vi "Autonomous Independent.vi"   [LabVIEW 2013]
doc: "This VI is called when autonomous begins, and will automatically be terminated when autonomous ends. You can carry out timed or sensor driven robot movement independently without needing to return to the caller."
uses:
  <vilib>/Rock Robotics/WPI/SafetyOutput/WPI_SafetyOutputConfigMenu.ctl
  <vilib>/Rock Robotics/WPI/Solenoid/WPI_SolenoidValue.ctl
  Robot Global Data.vi
  <vilib>/Rock Robotics/WPI/RobotDrive/WPI_RobotDriveGetSetRefNum.vi
  <vilib>/Rock Robotics/WPI/Solenoid/WPI_SolenoidSetEnum.vi
  <vilib>/Rock Robotics/WPI/RobotDrive/WPI_RobotDriveArcadeDrive_Standard(NoSaturation).vi
panel:
  # "Be sure to right-click and choose Data Operations>>Make Current Value default if you want to save the array values with the VI"
types:
  T1 = typedef "WPI_SafetyOutputConfigMenu.ctl" = enum16{"Enable", "Disable"}
  T2 = typedef "WPI_RobotDriveDevRef.ctl" = cluster{"DevStatus":errorcluster, "Motors[]":T3[], "Square Inputs":bool, "Max Output":dbl, "Isochronous":bool}
  T3 = typedef "WPI_MotorControlDeviceRef.ctl" = cluster{"DeviceStatus":errorcluster, "Type":enum16{"PWM", "CAN"}, "PWM":cluster{"Digital Module":T4, "PWM Channel":T5, "DeadBand":T6}, "CAN":cluster{"Device Number":u8, "Control Mode":T7, "Semaphore":T8, "Max Vout":dbl}, "Invert":bool, "TransformRef":T9, "InvTransformRef":T9}
  T4 = typedef "FPGA_TypedefDigitalModule.ctl" = enum16{"Digital Module 1", "Digital Module 2"}
  T5 = typedef "FPGA_DIOPWMChannel.ctl" = enum8{"PWM 1", "PWM 2", "PWM 3", "PWM 4", "PWM 5", "PWM 6", "PWM 7", "PWM 8", "PWM 9", "PWM 10", "Invalid"}
  T6 = typedef "WPI_PWMDeadband.ctl" = cluster{"Name":string, "maxPositivePwm":i32, "minPositivePwm":i32, "centerPwm":i32, "maxNegativePwm":i32, "minNegativePwm":i32, "angularRange":u16}
  T7 = typedef "WPI_CANJaguar_ControlMode.ctl" = enum8{"Percent VBus", "Current", "Speed", "Position", "Voltage"}
  T8 = typedef "Semaphore RefNum" = refnum<k1>
  T9 = typedef "WPI_PWMTransform_ConPane.ctl" = refnum<vi>
  T10 = typedef "WPI_EncoderDevRef.ctl" = cluster{"DevStatus":errorcluster, "EncoderIndex":T11, "CounterIndex":T12, "DistancePerCount":dbl, "Decoding Type":T13}
  T11 = typedef "FPGA_EncoderIdx.ctl" = enum8{"Enc 0", "Enc 1", "Enc 2", "Enc 3", "Invalid"}
  T12 = typedef "FPGA_CounterCtrSystemIndex.ctl" = enum8{"Ctr 0", "Ctr 1", "Ctr 2", "Ctr 3", "Ctr 4", "Ctr 5", "Ctr 6", "Ctr 7", "Invalid"}
  T13 = typedef "WPI_EncoderType.ctl" = enum16{"1x", "2x", "4x"}
  T14 = typedef "WPI_SolenoidDevRef.ctl" = cluster{"DevStatus":errorcluster, "Solenoid Module":T15, "Forward Solenoid Channel":T16, "Reverse Solenoid Channel":T16}
  T15 = typedef "FPGA_TypedefSolenoidModule.ctl" = enum16{"Solenoid Module 1", "Solenoid Module 2"}
  T16 = typedef "WPI_SolenoidChannel.ctl" = enum8{"Solenoid 1", "Solenoid 2", "Solenoid 3", "Solenoid 4", "Solenoid 5", "Solenoid 6", "Solenoid 7", "Solenoid 8", "Invalid"}
  T17 = typedef "WPI_DigitalInputDevRef.ctl" = cluster{"DevStatus":errorcluster, "DIO Channel":T18, "Digital Module":T4}
  T18 = typedef "FPGA_DIOChannel.ctl" = enum8{"DIO 1", "DIO 2", "DIO 3", "DIO 4", "DIO 5", "DIO 6", "DIO 7", "DIO 8", "DIO 9", "DIO 10", "DIO 11", "DIO 12", "DIO 13", "DIO 14", "Invalid"}
  T19 = typedef "WPI_SolenoidValue.ctl" = enum16{"Off", "On", "Forward", "Reverse"}
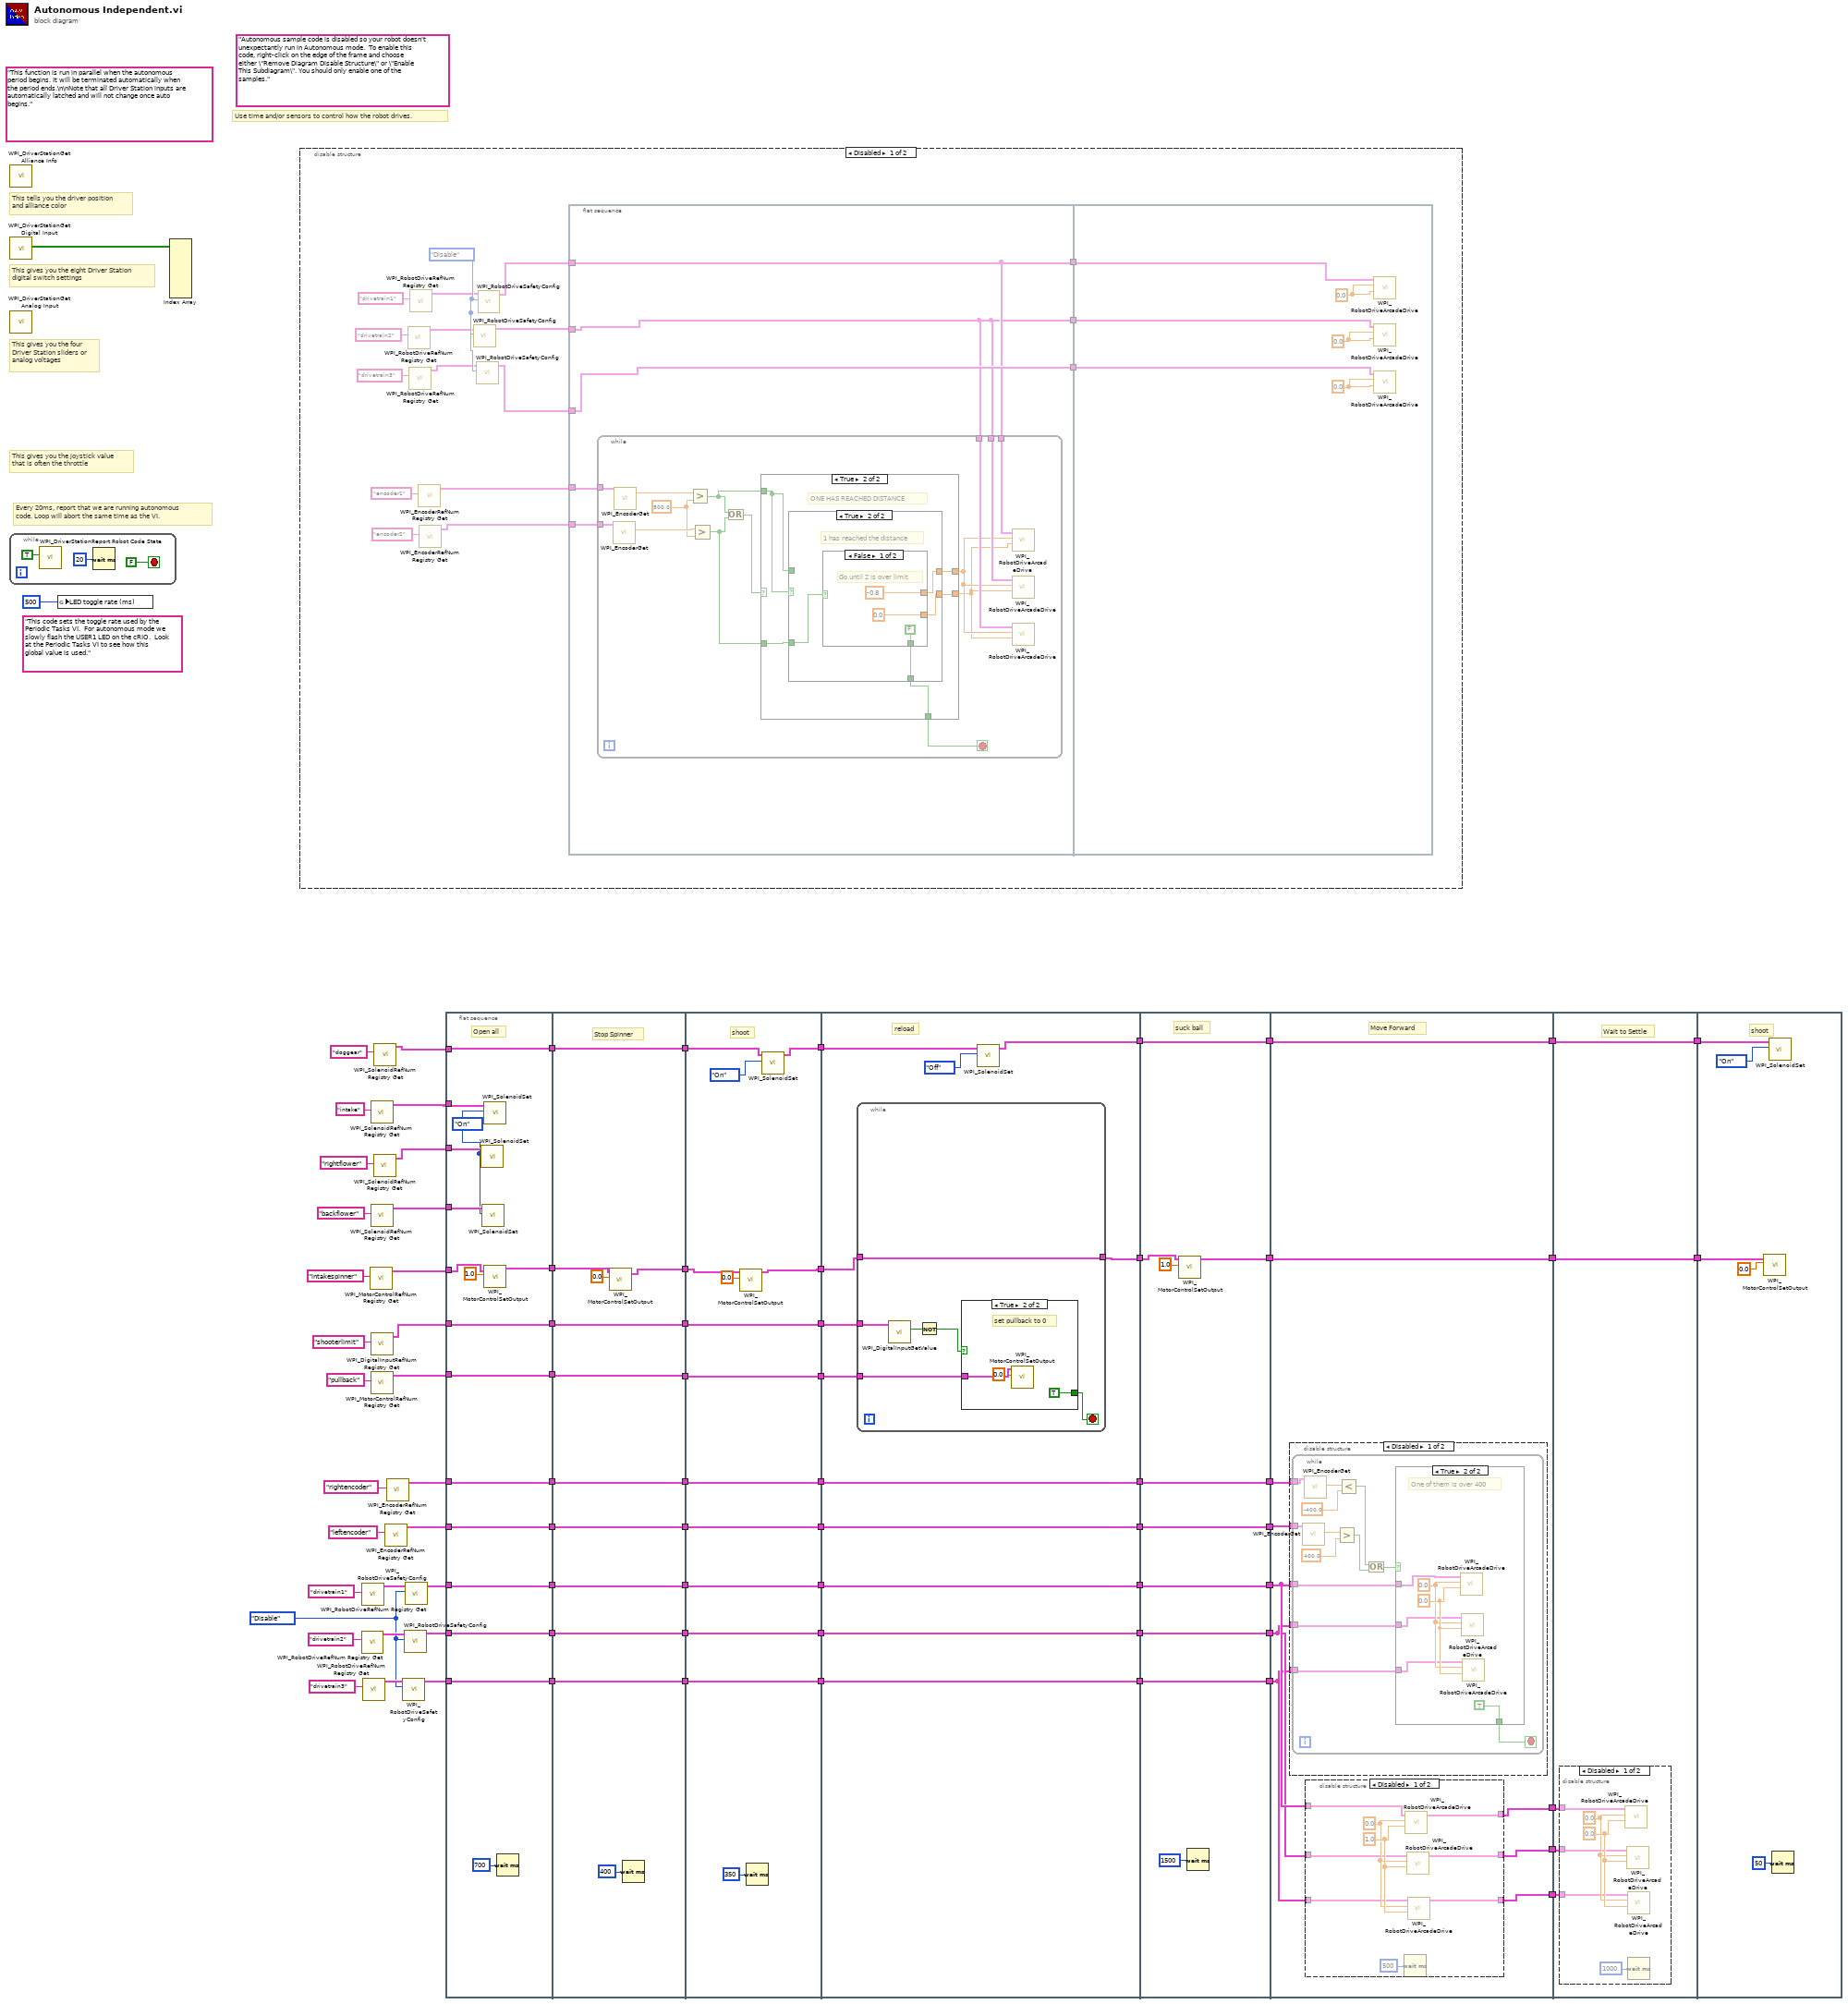
[diagram p0: block diagram]
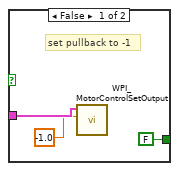
[diagram p2: hidden frame]
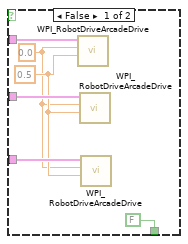
[diagram p4: hidden frame]
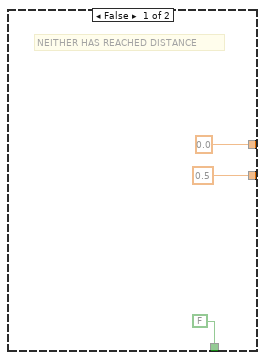
[diagram p7: hidden frame]
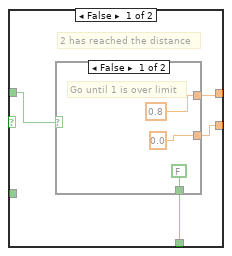
[diagram p8: hidden frame]
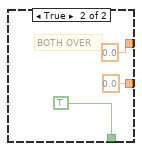
[diagram p9: hidden frame]
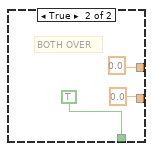
[diagram p10: hidden frame]
diagram:
  w38 = WPI_SafetyOutputConfigMenu."Disable" ("mode")
  (unwired) "This code sets the toggle rate used by the Periodic Tasks VI.  For autonomous mode we slowly flash the USER1 LED on the cRIO.  Look at the Periodic Tasks VI to see how this global value is used."
  (unwired) "Autonomous sample code is disabled so your robot doesn't unexpectantly run in Autonomous mode.  To enable this code, right-click on the edge of the frame and choose either \"Remove Diagram Disable Structure\" or \"Enable This Subdiagram\". You should only enable one of the samples."
  (unwired) "This function is run in parallel when the autonomous period begins. It will be terminated automatically when the period ends.\n\nNote that all Driver Station inputs are automatically latched and will not change once auto begins."
  # "Every 20ms, report that we are running autonomous\ncode. Loop will abort the same time as the VI."
  # "This gives you the joystick value\nthat is often the throttle"
  # "Use time and/or sensors to control how the robot drives."
  # "This tells you the driver position\nand alliance color"
  # "This gives you the eight Driver Station\ndigital switch settings"
  # "This gives you the four\nDriver Station sliders or\nanalog voltages"
  n1 = while {
    stop <- FALSE stop-if-true
    n2 = call <vilib>:"WPI_DriverStationReport Robot Code State.vi"("Autonomous"=TRUE) -> ()  [unwired: 10 in, 1 out]
    n3 = Wait (ms)(milliseconds to wait=u32 20) -> ()  [unwired: 1 out]
  }
  n4 = call <vilib>:"WPI_DriverStationGet Alliance Info.vi"() -> ()  [unwired: 12 out]
  n5 = call <vilib>:"WPI_DriverStationGet Digital Input.vi"() -> ("Driver Station Digital Input (1-8)"=w78:bool[])  [unwired: 11 out]
  n6 = call <vilib>:"WPI_DriverStationGet Analog Input.vi"() -> ()  [unwired: 12 out]
  n7 = global write "Robot Global Data.vi" "LED toggle rate (ms)"(u32 500 ("LED ms toggle rate")) -> ()
  n8 = Index Array(array=w78) -> ()  [unwired: 8 in, 8 out]
  n9 = disable-structure shown="Disabled" {
    frame Disabled {
      w92 = WPI_SafetyOutputConfigMenu."Disable" ("mode")
      n10 = call <vilib>:"WPI_RobotDriveRefNum Registry Get.vi"("refnum name"="drivetrain2") -> ("RobotDriveDevRef"=w90:T2)  [unwired: 9 in, 1 out]
      n11 = call <vilib>:"WPI_RobotDriveRefNum Registry Get.vi"("refnum name"="drivetrain3") -> ("RobotDriveDevRef"=w89:T2)  [unwired: 9 in, 1 out]
      n12 = call <vilib>:"WPI_RobotDriveRefNum Registry Get.vi"("refnum name"="drivetrain1") -> ("RobotDriveDevRef"=w91:T2)  [unwired: 9 in, 1 out]
      n13 = call <vilib>:"WPI_EncoderRefNum Registry Get.vi"("refnum name"="encoder1") -> ("EncoderDevRef"=w85:T10)  [unwired: 9 in, 1 out]
      n14 = call <vilib>:"WPI_EncoderRefNum Registry Get.vi"("refnum name"="encoder2") -> ("EncoderDevRef"=w84:T10)  [unwired: 9 in, 1 out]
      n15 = call <vilib>:"WPI_RobotDriveSafetyConfig.vi"("mode"=w92, "RobotDriveDevRef"=w90) -> ("RobotDriveDevRef"=w87:T2)  [unwired: 8 in, 1 out]
      n16 = call <vilib>:"WPI_RobotDriveSafetyConfig.vi"("mode"=w92, "RobotDriveDevRef"=w89) -> ("RobotDriveDevRef"=w86:T2)  [unwired: 8 in, 1 out]
      n17 = call <vilib>:"WPI_RobotDriveSafetyConfig.vi"("mode"=w92, "RobotDriveDevRef"=w91) -> ("RobotDriveDevRef"=w88:T2)  [unwired: 8 in, 1 out]
      n18 = flat-sequence {
        tunnel: w88 -> [w100]
        tunnel: w87 -> [w99]
        tunnel: w86 -> [w103]
        tunnel: [w100] -> w98
        tunnel: [w99] -> w97
        tunnel: [w103] -> w96
        tunnel: w85 -> [w102]
        tunnel: w84 -> [w101]
        tunnel: w98 -> [w151]
        tunnel: w97 -> [w150]
        tunnel: w96 -> [w149]
        frame #0 {
          n19 = while {
            tunnel: w102 -> [w117]
            tunnel: w101 -> [w116]
            tunnel: w100 -> [w109]
            tunnel: w99 -> [w108]
            tunnel: w99 -> [w107]
            stop <- w111 stop-if-true
            w113 = 500.0 ("y")
            n20 = call <vilib>:"WPI_EncoderGet.vi"("EncoderDevRef"=w116) -> ("Distance"=w114:dbl)  [unwired: 5 in, 5 out]
            n21 = call <vilib>:"WPI_EncoderGet.vi"("EncoderDevRef"=w117) -> ("Distance"=w115:dbl)  [unwired: 5 in, 5 out]
            n22 = Greater?(x=w115, y=w113) -> (0:w110:bool)
            n23 = Greater?(x=w114, y=w113) -> (0:w106:bool)
            n24 = Or(x=w110, y=w106) -> (x .or. y?=w112:bool)
            n25 = case shown="True" w112 {
              tunnel: [FALSE w123] -> w111
              tunnel: w110 -> [_ w124]
              tunnel: w106 -> [_ w125]
              tunnel: [0.0 ("y") w122] -> w105
              tunnel: [0.5 ("y") w121] -> w104
              frame False {
                # "NEITHER HAS REACHED DISTANCE"
              }
              frame True {
                # "ONE HAS REACHED DISTANCE"
                n26 = case shown="True" w124 {
                  tunnel: w125 -> [_ w139]
                  tunnel: w124 -> [w129 _]
                  tunnel: [w128 w138] -> w123
                  tunnel: [w127 w137] -> w122
                  tunnel: [w126 w136] -> w121
                  frame False {
                    # "2 has reached the distance"
                    n27 = case shown="False" w129 {
                      tunnel: [FALSE TRUE] -> w128
                      tunnel: [0.8 ("y") 0.0 ("y")] -> w127
                      tunnel: [0.0 ("y") 0.0 ("y")] -> w126
                      frame False {
                        # "Go until 1 is over limit"
                      }
                      frame True {
                        # "BOTH OVER"
                      }
                    }
                  }
                  frame True {
                    # "1 has reached the distance"
                    n28 = case shown="False" w139 {
                      tunnel: [FALSE TRUE] -> w138
                      tunnel: [-0.8 ("y") 0.0 ("y")] -> w137
                      tunnel: [0.0 ("y") 0.0 ("y")] -> w136
                      frame False {
                        # "Go until 2 is over limit"
                      }
                      frame True {
                        # "BOTH OVER"
                      }
                    }
                  }
                }
              }
            }
            n29 = call-poly <vilib>:"WPI_RobotDriveArcadeDrive.vi"("Y axis value"=w104, "X axis value"=w105, "RobotDriveDevRef"=w109) -> ()  [unwired: 6 in, 3 out]
            n30 = call-poly <vilib>:"WPI_RobotDriveArcadeDrive.vi"("Y axis value"=w104, "X axis value"=w105, "RobotDriveDevRef"=w108) -> ()  [unwired: 6 in, 3 out]
            n31 = call-poly <vilib>:"WPI_RobotDriveArcadeDrive.vi"("Y axis value"=w104, "X axis value"=w105, "RobotDriveDevRef"=w107) -> ()  [unwired: 6 in, 3 out]
          }
        }
        frame #1 {
          w146 = 0.0 ("Y axis value")
          w147 = 0.0 ("Y axis value")
          w148 = 0.0 ("Y axis value")
          n32 = call-poly <vilib>:"WPI_RobotDriveArcadeDrive.vi"("Y axis value"=w148, "X axis value"=w148, "RobotDriveDevRef"=w151) -> ()  [unwired: 6 in, 3 out]
          n33 = call-poly <vilib>:"WPI_RobotDriveArcadeDrive.vi"("Y axis value"=w147, "X axis value"=w147, "RobotDriveDevRef"=w150) -> ()  [unwired: 6 in, 3 out]
          n34 = call-poly <vilib>:"WPI_RobotDriveArcadeDrive.vi"("Y axis value"=w146, "X axis value"=w146, "RobotDriveDevRef"=w149) -> ()  [unwired: 6 in, 3 out]
        }
      }
    }
    frame Enabled {
    }
  }
  n35 = call <vilib>:"WPI_RobotDriveRefNum Registry Get.vi"("refnum name"="drivetrain2") -> ("RobotDriveDevRef"=w40:T2)  [unwired: 9 in, 1 out]
  n36 = call <vilib>:"WPI_RobotDriveRefNum Registry Get.vi"("refnum name"="drivetrain1") -> ("RobotDriveDevRef"=w41:T2)  [unwired: 9 in, 1 out]
  n37 = call <vilib>:"WPI_RobotDriveRefNum Registry Get.vi"("refnum name"="drivetrain3") -> ("RobotDriveDevRef"=w39:T2)  [unwired: 9 in, 1 out]
  n38 = call <vilib>:"WPI_MotorControlRefNum Registry Get.vi"("refnum name"="intakespinner") -> ("MotorControlDevRef"=w66:T3)  [unwired: 9 in, 1 out]
  n39 = call <vilib>:"WPI_SolenoidRefNum Registry Get.vi"("refnum name"="intake") -> ("SolenoidDevRef"=w70:T14)  [unwired: 9 in, 1 out]
  n40 = call <vilib>:"WPI_SolenoidRefNum Registry Get.vi"("refnum name"="backflower") -> ("SolenoidDevRef"=w68:T14)  [unwired: 9 in, 1 out]
  n41 = call <vilib>:"WPI_DigitalInputRefNum Registry Get.vi"("refnum name"="shooterlimit") -> ("DigitalInputDevRef"=w63:T17)  [unwired: 9 in, 1 out]
  n42 = call <vilib>:"WPI_MotorControlRefNum Registry Get.vi"("refnum name"="pullback") -> ("MotorControlDevRef"=w60:T3)  [unwired: 9 in, 1 out]
  n43 = call <vilib>:"WPI_SolenoidRefNum Registry Get.vi"("refnum name"="rightflower") -> ("SolenoidDevRef"=w69:T14)  [unwired: 9 in, 1 out]
  n44 = call <vilib>:"WPI_SolenoidRefNum Registry Get.vi"("refnum name"="doggear") -> ("SolenoidDevRef"=w75:T14)  [unwired: 9 in, 1 out]
  n45 = call <vilib>:"WPI_EncoderRefNum Registry Get.vi"("refnum name"="leftencoder") -> ("EncoderDevRef"=w34:T10)  [unwired: 9 in, 1 out]
  n46 = call <vilib>:"WPI_EncoderRefNum Registry Get.vi"("refnum name"="rightencoder") -> ("EncoderDevRef"=w36:T10)  [unwired: 9 in, 1 out]
  n47 = call <vilib>:"WPI_RobotDriveSafetyConfig.vi"("mode"=w38, "RobotDriveDevRef"=w39) -> ("RobotDriveDevRef"=w12:T2)  [unwired: 8 in, 1 out]
  n48 = call <vilib>:"WPI_RobotDriveSafetyConfig.vi"("mode"=w38, "RobotDriveDevRef"=w40) -> ("RobotDriveDevRef"=w22:T2)  [unwired: 8 in, 1 out]
  n49 = call <vilib>:"WPI_RobotDriveSafetyConfig.vi"("mode"=w38, "RobotDriveDevRef"=w41) -> ("RobotDriveDevRef"=w24:T2)  [unwired: 8 in, 1 out]
  n50 = flat-sequence {
    tunnel: w75 -> [w167]
    tunnel: [w167] -> w74
    tunnel: w70 -> [w166]
    tunnel: w69 -> [w165]
    tunnel: w68 -> [w164]
    tunnel: w66 -> [w161]
    tunnel: [w159] -> w65
    tunnel: w63 -> [w158]
    tunnel: [w158] -> w62
    tunnel: w60 -> [w157]
    tunnel: [w157] -> w59
    tunnel: [w156] -> w37
    tunnel: w36 -> [w156]
    tunnel: [w155] -> w35
    tunnel: w34 -> [w155]
    tunnel: [w154] -> w25
    tunnel: w24 -> [w154]
    tunnel: [w153] -> w23
    tunnel: w22 -> [w153]
    tunnel: [w152] -> w13
    tunnel: w12 -> [w152]
    tunnel: w74 -> [w173]
    tunnel: w65 -> [w179]
    tunnel: [w176] -> w56
    tunnel: [w175] -> w54
    tunnel: w62 -> [w175]
    tunnel: w59 -> [w174]
    tunnel: [w174] -> w52
    tunnel: [w173] -> w49
    tunnel: w37 -> [w171]
    tunnel: w35 -> [w172]
    tunnel: [w172] -> w31
    tunnel: [w171] -> w28
    tunnel: w25 -> [w170]
    tunnel: w23 -> [w169]
    tunnel: [w170] -> w18
    tunnel: [w169] -> w14
    tunnel: w13 -> [w168]
    tunnel: [w168] -> w8
    tunnel: w56 -> [w191]
    tunnel: [w190] -> w55
    tunnel: w54 -> [w193]
    tunnel: [w193] -> w53
    tunnel: w52 -> [w192]
    tunnel: [w192] -> w51
    tunnel: [w186] -> w50
    tunnel: w49 -> [w185]
    tunnel: [w184] -> w32
    tunnel: w31 -> [w184]
    tunnel: [w183] -> w29
    tunnel: w28 -> [w183]
    tunnel: [w182] -> w19
    tunnel: w18 -> [w182]
    tunnel: [w181] -> w15
    tunnel: w14 -> [w181]
    tunnel: [w180] -> w9
    tunnel: w8 -> [w180]
    tunnel: w55 -> [w202]
    tunnel: w53 -> [w205]
    tunnel: w51 -> [w204]
    tunnel: [w203] -> w58
    tunnel: [w200] -> w57
    tunnel: w50 -> [w199]
    tunnel: [w198] -> w33
    tunnel: w32 -> [w198]
    tunnel: [w197] -> w30
    tunnel: w29 -> [w197]
    tunnel: [w196] -> w20
    tunnel: w19 -> [w196]
    tunnel: [w195] -> w16
    tunnel: w15 -> [w195]
    tunnel: [w194] -> w10
    tunnel: w9 -> [w194]
    tunnel: [w227] -> w46
    tunnel: [w223] -> w45
    tunnel: w57 -> [w227]
    tunnel: w58 -> [w224]
    tunnel: w33 -> [w221]
    tunnel: w30 -> [w222]
    tunnel: [w222] -> w27
    tunnel: [w221] -> w26
    tunnel: [w220] -> w21
    tunnel: w20 -> [w220]
    tunnel: [w219] -> w17
    tunnel: w16 -> [w219]
    tunnel: [w218] -> w11
    tunnel: w10 -> [w218]
    tunnel: w46 -> [w237]
    tunnel: [w237] -> w7
    tunnel: w45 -> [w236]
    tunnel: [w236] -> w5
    tunnel: w27 -> [w235]
    tunnel: w26 -> [w234]
    tunnel: w21 -> [w233]
    tunnel: w17 -> [w232]
    tunnel: w11 -> [w231]
    tunnel: [w230] -> w3
    tunnel: [w229] -> w2
    tunnel: [w228] -> w1
    tunnel: w7 -> [w281]
    tunnel: [w281] -> w6
    tunnel: w5 -> [w280]
    tunnel: [w280] -> w4
    tunnel: w3 -> [w279]
    tunnel: w2 -> [w278]
    tunnel: w1 -> [w277]
    tunnel: w6 -> [w290]
    tunnel: w4 -> [w288]
    frame #0 {
      w163 = WPI_SolenoidValue."On" ("Value")
      # "Open all"
      n51 = call-poly <vilib>:"WPI_SolenoidSet.vi"("Value"=w163, "SolenoidDevRef"=w165) -> ()  [unwired: 8 in, 2 out]
      n52 = call-poly <vilib>:"WPI_SolenoidSet.vi"("Value"=w163, "SolenoidDevRef"=w164) -> ()  [unwired: 8 in, 2 out]
      n53 = call-poly <vilib>:"WPI_SolenoidSet.vi"("Value"=w163, "SolenoidDevRef"=w166) -> ()  [unwired: 8 in, 2 out]
      n54 = call <vilib>:"WPI_MotorControlSetOutput.vi"("Output"=1.0, "MotorControlDevRef"=w161) -> ("MotorControlDevRef"=w159:T3)  [unwired: 7 in, 2 out]
      n55 = Wait (ms)(milliseconds to wait=u32 700) -> ()  [unwired: 1 out]
    }
    frame #1 {
      # "Stop Spinner"
      n56 = call <vilib>:"WPI_MotorControlSetOutput.vi"("Output"=0.0, "MotorControlDevRef"=w179) -> ("MotorControlDevRef"=w176:T3)  [unwired: 7 in, 2 out]
      n57 = Wait (ms)(milliseconds to wait=u32 400) -> ()  [unwired: 1 out]
    }
    frame #2 {
      # "shoot"
      n58 = call <vilib>:"WPI_MotorControlSetOutput.vi"("Output"=0.0, "MotorControlDevRef"=w191) -> ("MotorControlDevRef"=w190:T3)  [unwired: 7 in, 2 out]
      n59 = Wait (ms)(milliseconds to wait=u32 350) -> ()  [unwired: 1 out]
      n60 = call-poly <vilib>:"WPI_SolenoidSet.vi"("Value"=WPI_SolenoidValue."On", "SolenoidDevRef"=w185) -> ("SolenoidDevRef"=w186:T14)  [unwired: 8 in, 1 out]
    }
    frame #3 {
      # "reload"
      n61 = while {
        tunnel: w205 -> [w211]
        tunnel: w204 -> [w208]
        tunnel: [w206] -> w203
        tunnel: w202 -> [w206]
        stop <- w207 stop-if-true
        n62 = call <vilib>:"WPI_DigitalInputGetValue.vi"("DigitalInputDevRef"=w211) -> ("Value"=w210:bool)  [unwired: 8 in, 2 out]
        n63 = Not(x=w210) -> (.not. x?=w209:bool)
        n64 = case shown="True" w209 {
          tunnel: w208 -> [w214 w217]
          tunnel: [FALSE TRUE] -> w207
          frame False {
            # "set pullback to -1"
            n65 = call <vilib>:"WPI_MotorControlSetOutput.vi"("Output"=-1.0, "MotorControlDevRef"=w214) -> ()  [unwired: 7 in, 3 out]
          }
          frame True {
            # "set pullback to 0"
            n66 = call <vilib>:"WPI_MotorControlSetOutput.vi"("Output"=0.0, "MotorControlDevRef"=w217) -> ()  [unwired: 7 in, 3 out]
          }
        }
      }
      n67 = call-poly <vilib>:"WPI_SolenoidSet.vi"("Value"=WPI_SolenoidValue."Off", "SolenoidDevRef"=w199) -> ("SolenoidDevRef"=w200:T14)  [unwired: 8 in, 1 out]
    }
    frame #4 {
      # "suck ball"
      n68 = call <vilib>:"WPI_MotorControlSetOutput.vi"("Output"=1.0, "MotorControlDevRef"=w224) -> ("MotorControlDevRef"=w223:T3)  [unwired: 7 in, 2 out]
      n69 = Wait (ms)(milliseconds to wait=u32 1500) -> ()  [unwired: 1 out]
    }
    frame #5 {
      # "Move Forward"
      n70 = disable-structure shown="Disabled" {
        disable-tunnel: w235 -> [w251 _]
        disable-tunnel: w234 -> [w250 _]
        disable-tunnel: w233 -> [w249 _]
        disable-tunnel: w232 -> [w248 _]
        disable-tunnel: w231 -> [w247 _]
        frame Disabled {
          n71 = while {
            tunnel: w251 -> [w264]
            tunnel: w250 -> [w263]
            tunnel: w249 -> [w260]
            tunnel: w248 -> [w259]
            tunnel: w247 -> [w258]
            stop <- w261 stop-if-true
            n72 = call <vilib>:"WPI_EncoderGet.vi"("EncoderDevRef"=w263) -> ("Distance"=w254:dbl)  [unwired: 5 in, 5 out]
            n73 = call <vilib>:"WPI_EncoderGet.vi"("EncoderDevRef"=w264) -> ("Distance"=w257:dbl)  [unwired: 5 in, 5 out]
            n74 = Greater?(x=w254, y=400.0) -> (0:w252:bool)
            n75 = Less?(x=w257, y=-400.0) -> (x < y?=w255:bool)
            n76 = Or(x=w255, y=w252) -> (x .or. y?=w262:bool)
            n77 = case shown="True" w262 {
              tunnel: [FALSE TRUE] -> w261
              tunnel: w260 -> [w269 w273]
              tunnel: w259 -> [w268 w272]
              tunnel: w258 -> [w267 w271]
              frame False {
                w265 = 0.0 ("Y axis value")
                w266 = 0.5 ("Y axis value")
                n78 = call-poly <vilib>:"WPI_RobotDriveArcadeDrive.vi"("Y axis value"=w266, "X axis value"=w265, "RobotDriveDevRef"=w269) -> ()  [unwired: 6 in, 3 out]
                n79 = call-poly <vilib>:"WPI_RobotDriveArcadeDrive.vi"("Y axis value"=w266, "X axis value"=w265, "RobotDriveDevRef"=w268) -> ()  [unwired: 6 in, 3 out]
                n80 = call-poly <vilib>:"WPI_RobotDriveArcadeDrive.vi"("Y axis value"=w266, "X axis value"=w265, "RobotDriveDevRef"=w267) -> ()  [unwired: 6 in, 3 out]
              }
              frame True {
                w274 = 0.0 ("Y axis value")
                w275 = 0.0 ("Y axis value")
                # "One of them is over 400"
                n81 = call-poly <vilib>:"WPI_RobotDriveArcadeDrive.vi"("Y axis value"=w275, "X axis value"=w274, "RobotDriveDevRef"=w273) -> ()  [unwired: 6 in, 3 out]
                n82 = call-poly <vilib>:"WPI_RobotDriveArcadeDrive.vi"("Y axis value"=w275, "X axis value"=w274, "RobotDriveDevRef"=w272) -> ()  [unwired: 6 in, 3 out]
                n83 = call-poly <vilib>:"WPI_RobotDriveArcadeDrive.vi"("Y axis value"=w275, "X axis value"=w274, "RobotDriveDevRef"=w271) -> ()  [unwired: 6 in, 3 out]
              }
            }
          }
        }
        frame Enabled {
        }
      }
      n84 = disable-structure shown="Disabled" {
        disable-tunnel: w233 -> [w243 _]
        disable-tunnel: w232 -> [w242 _]
        disable-tunnel: w231 -> [w241 _]
        disable-tunnel: [w240 _] -> w230
        disable-tunnel: [w239 _] -> w229
        disable-tunnel: [w238 _] -> w228
        frame Disabled {
          w244 = 0.0 ("Y axis value")
          w245 = 1.0 ("Y axis value")
          n85 = Wait (ms)(milliseconds to wait=u32 500) -> ()  [unwired: 1 out]
          n86 = call-poly <vilib>:"WPI_RobotDriveArcadeDrive.vi"("Y axis value"=w245, "X axis value"=w244, "RobotDriveDevRef"=w243) -> ("RobotDriveDevRef"=w240:T2)  [unwired: 6 in, 2 out]
          n87 = call-poly <vilib>:"WPI_RobotDriveArcadeDrive.vi"("Y axis value"=w245, "X axis value"=w244, "RobotDriveDevRef"=w242) -> ("RobotDriveDevRef"=w239:T2)  [unwired: 6 in, 2 out]
          n88 = call-poly <vilib>:"WPI_RobotDriveArcadeDrive.vi"("Y axis value"=w245, "X axis value"=w244, "RobotDriveDevRef"=w241) -> ("RobotDriveDevRef"=w238:T2)  [unwired: 6 in, 2 out]
        }
        frame Enabled {
        }
      }
    }
    frame #6 {
      # "Wait to Settle"
      n89 = disable-structure shown="Disabled" {
        disable-tunnel: w279 -> [w284 _]
        disable-tunnel: w278 -> [w283 _]
        disable-tunnel: w277 -> [w282 _]
        frame Disabled {
          w285 = 0.0 ("Y axis value")
          w286 = 0.0 ("Y axis value")
          n90 = call-poly <vilib>:"WPI_RobotDriveArcadeDrive.vi"("Y axis value"=w286, "X axis value"=w285, "RobotDriveDevRef"=w284) -> ()  [unwired: 6 in, 3 out]
          n91 = call-poly <vilib>:"WPI_RobotDriveArcadeDrive.vi"("Y axis value"=w286, "X axis value"=w285, "RobotDriveDevRef"=w283) -> ()  [unwired: 6 in, 3 out]
          n92 = call-poly <vilib>:"WPI_RobotDriveArcadeDrive.vi"("Y axis value"=w286, "X axis value"=w285, "RobotDriveDevRef"=w282) -> ()  [unwired: 6 in, 3 out]
          n93 = Wait (ms)(milliseconds to wait=u32 1000) -> ()  [unwired: 1 out]
        }
        frame Enabled {
        }
      }
    }
    frame #7 {
      # "shoot"
      n94 = call <vilib>:"WPI_MotorControlSetOutput.vi"("Output"=0.0, "MotorControlDevRef"=w288) -> ()  [unwired: 7 in, 3 out]
      n95 = call-poly <vilib>:"WPI_SolenoidSet.vi"("Value"=WPI_SolenoidValue."On", "SolenoidDevRef"=w290) -> ()  [unwired: 8 in, 2 out]
      n96 = Wait (ms)(milliseconds to wait=u32 50) -> ()  [unwired: 1 out]
    }
  }
